vi "Get Handle.vi"(8 "error in (no error)":errorcluster, 10 "Symbol Name":string, 11 "TwinCAT ADS in":refnum<class "TwinCAT ADS.lvclass">) -> (0 "error out":errorcluster, 2 "Handle":i32=-1, 3 "TwinCAT ADS out":refnum<class "TwinCAT ADS.lvclass">)   [LabVIEW 2018, in "TwinCAT ADS.lvclass"]
uses:
  TwinCAT ADS.lvclass
  TwinCAT ADS.lvclass/TwinCAT ADS.ctl
  TwinCAT.Ads
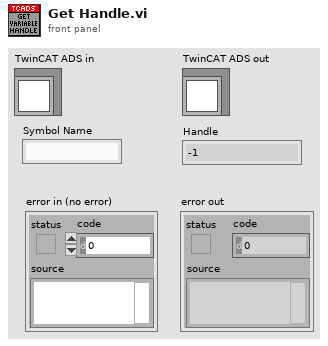
[diagram p1: front panel]
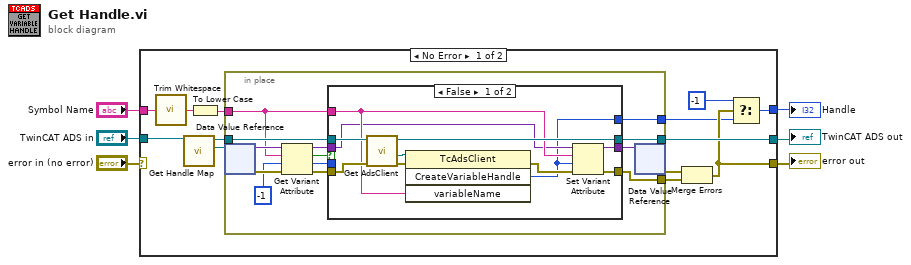
[diagram p0: block diagram]
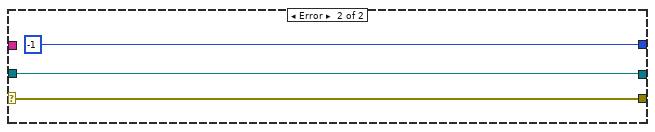
[diagram p3: hidden frame]
diagram:
  n1 = case shown="No Error" "error in (no error)" {
    selector: "error in (no error)" -> [_ w49]
    tunnel: "TwinCAT ADS in" -> [w19 w50]
    tunnel: "Symbol Name" -> [w15 _]
    tunnel: [w7 -1 ("CreateVariableHandle")] -> w4
    tunnel: [w13 w50] -> w3
    tunnel: [w9 w49] -> w1
    frame No Error {
      n2 = call <vilib>:"Trim Whitespace.vi"("string"=w15) -> ("trimmed string"=w16:string)  [unwired: 1 in]
      n3 = call "Get Handle Map.vi"("TwinCAT ADS in"=w19) -> ("Handle Map"=w18:refnum<data-value>, "TwinCAT ADS out"=w14:refnum<class "TwinCAT ADS.lvclass">)  [unwired: 8 in, 1 out]
      n4 = To Lower Case(string=w16) -> (all lower case string=w17:string)
      n5 = in-place {
        in-place-border: w17 -> [w24]
        in-place-border: w14 -> [w32]
        in-place-border: [w23] -> w8
        in-place-border: [w22] -> w13
        in-place-border: [w20] -> w11
        n6 = in-place-dvr #1(w18) -> (w31:variant, w30:errorcluster)
        n7 = Get Variant Attribute(Variant=w31, name=w24, default value (empty Variant)=-1 ("CreateVariableHandle"), error in=w30) -> (duplicate Variant=w26:variant, found=w28:bool, value=w27:i32, error out=w25:errorcluster)
        n8 = case shown="False" w28 {
          tunnel: w27 -> [_ w45]
          tunnel: w32 -> [w41 w47]
          tunnel: w26 -> [w37 w44]
          tunnel: w25 -> [w40 w46]
          tunnel: w24 -> [w38 _]
          tunnel: [w39 w47] -> w22
          tunnel: [w34 w46] -> w20
          tunnel: [w33 w45] -> w23
          tunnel: [w36 w44] -> w21
          frame False {
            n9 = call "Get AdsClient.vi"("error in (no error)"=w40, "TwinCAT ADS in"=w41) -> ("error out"=w43:errorcluster, ".NET TcAdsClient"=w42:refnum<k24>, "TwinCAT ADS out"=w39:refnum<class "TwinCAT ADS.lvclass">)  [unwired: 7 in]
            n10 = invoke class="TcAdsClient" method="CreateVariableHandle"(reference=w42, error in=w43, "variableName"=w38) -> (error out=w35:errorcluster, "CreateVariableHandle"=w33:i32)  [unwired: 1 in, 2 out]
            n11 = Set Variant Attribute(Variant=w37, name=w38, value=w33, error in=w35) -> (Variant out=w36:variant, error out=w34:errorcluster)  [unwired: 1 out]
          }
          frame True {
          }
        }
        n12 = in-place-dvr #1(w21) -> (w12:errorcluster)  [unwired: 1 out]
      }
      n13 = Merge Errors(w12, w11) -> (w9:errorcluster)
      n14 = Select(t=-1 ("CreateVariableHandle"), s=w9, f=w8) -> (s? t:f=w7:i32)
    }
    frame Error {
    }
  }
  "error out" <- w1
  "TwinCAT ADS out" <- w3
  "Handle" <- w4
